vi "Global 1.vi"() -> ()   [LabVIEW 2011]
panel:
  out "Flip Axises?":bool
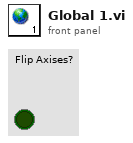
[diagram p1: front panel]
diagram:
